vi "handle_kf.vi"(6 "Reset":bool, 7 "Parameters":T2={"Stimulus"={"Type"=enum."Off", "Phase"=0.0, "Amplitude"=[], "Injection point"=enum."Total pose", "Closed loop"=FALSE, "Offset"=[], "Tip -> world"=FALSE, "Frequency"=0.0, "Length"=0.0}, "Goal Filter A"={"Speedup max"=0.0, "Speedup thresh"=0.0, "Speedup nonlin"=0.0, "Filters"=[]}, "Mode controls"={"Hold"=FALSE, "Cancellation"=FALSE, "Goal filter"=FALSE, "Trigger"=FALSE}, "Manipulator type"=enum."Current piezo", "Manipulator calibration"={"Tool offsets"=[[0.0, 0.0, 36200.0]], "Handle light calibration"=[], "Base pivots"=[], "Output pivots"=[], "Length center"=0.0, "Workspace height"=[], "Workspace diameter"=[0.0, 0.0, 36200.0], "Stack travel"=400.0, "Saturation pos"=375.0, "Inverse filters"=[], "Strut length"=0.0}, "Network"={"Remote Host"="", "Send Status"=FALSE, "Send Port"=0, "Recv Commands"=FALSE, "Recv Port"=0}, "Goal Filter B"={"Speedup max"=0.0, "Speedup thresh"=0.0, "Speedup nonlin"=0.0, "Filters"=[]}, "Cancellation"={"KP"={"XY"=0.0, "Rxy"=0.0, "Z"=0.0, "Rz"=0.0}, "KI"=0.0, "KD"={"XY"=0.0, "Rxy"=0.0, "Z"=0.0, "Rz"=0.0}, "Max vel"=20.0, "Max acc"=0.001, "Int error limit"=3.0, "RCM gain"=0.0, "Bypass"=FALSE, "Degraded gain"=0.0}, "Transition time"=0.0, "Estimation"={"Link"={"Measure noise"=[], "Process noise"=[], "Alt process noise"=[], "Alt turnoff cycles"=20, "Innovation limit"=[], "Residue threshold"=0.0, "Enable"=FALSE}, "Handle"={"Measure noise"=[], "Process noise"=[], "State limits"=[], "Innovation limit"=[], "Prediction Lookahead"=0.0, "Enable"=FALSE}}} {"Transition time" format="%_3f"; "Cancellation"."Degraded gain" min=0 max=1 step=0.1 format="%#_3p"; "Cancellation"."RCM gain" min=0 max=1 step=0.1 format="%#_3p"; "Cancellation"."KD"."Rz" min=-1 max=1 step=0.01 format="%#_3p"; "Cancellation"."KD"."Rxy" min=-1 max=1 step=0.01 format="%#_3p"; "Cancellation"."KD"."Z" min=-1 max=1 step=0.01 format="%#_3p"; "Cancellation"."KD"."XY" min=-1 max=1 step=0.01 format="%#_3p"; "Cancellation"."KI" min=0 max=1 step=0.01 format="%#_3p"; "Cancellation"."KP"."Rz" min=-1 max=1 step=0.01 format="%#_3p"; "Cancellation"."KP"."Rxy" min=-1 max=1 step=0.01 format="%#_3p"; "Cancellation"."KP"."Z" min=-1 max=1 step=0.01 format="%#_3p"; "Cancellation"."KP"."XY" min=-1 max=1 step=0.01 format="%#_3p"; "Cancellation"."Max acc" format="%#_3p"; "Goal Filter B"."Filters"."V limit range" format="%_3p"; "Goal Filter B"."Filters"."V limit" format="%_3p"; "Goal Filter B"."Filters"."Upper Q" format="%_3f"; "Goal Filter B"."Filters"."Upper Fc" format="%_3p"; "Goal Filter B"."Filters"."Lower Q" format="%_3f"; "Goal Filter B"."Filters"."Scale factor" format="%_3f"; "Goal Filter B"."Filters"."Lower Fc" format="%_3p"; "Goal Filter B"."Speedup nonlin" format="%_3p"; "Goal Filter B"."Speedup thresh" format="%_3p"; "Goal Filter B"."Speedup max" format="%_3p"; "Manipulator calibration"."Strut length" format="%#_4p"; "Manipulator calibration"."Saturation pos" format="%#.1f"; "Manipulator calibration"."Stack travel" format="%#.1f"; "Manipulator calibration"."Length center" format="%#_4p"; "Manipulator calibration"."Output pivots" format="%#_6f"; "Manipulator calibration"."Base pivots" format="%#_6f"; "Manipulator calibration"."Handle light calibration" format="%#.1f"; "Goal Filter A"."Filters"."V limit range" format="%_3p"; "Goal Filter A"."Filters"."V limit" format="%_3p"; "Goal Filter A"."Filters"."Upper Q" format="%_3f"; "Goal Filter A"."Filters"."Upper Fc" format="%_3p"; "Goal Filter A"."Filters"."Lower Q" format="%_3f"; "Goal Filter A"."Filters"."Scale factor" format="%_3f"; "Goal Filter A"."Filters"."Lower Fc" format="%_3p"; "Goal Filter A"."Speedup nonlin" format="%_3p"; "Goal Filter A"."Speedup thresh" format="%_3p"; "Goal Filter A"."Speedup max" format="%_3p"; "Stimulus"."Length" min=0.0 max=100.0 step=100.0 format="%#_4p"; "Stimulus"."Frequency" min=0.0 step=100.0 format="%#_4g"; "Stimulus"."Offset" format="%#_3p"; "Stimulus"."Amplitude" format="%#_3p"; "Stimulus"."Phase" min=-180.0 max=360.0 step=100.0 format="%#.2f"}, 11 "Handle Pose":T1) -> (1 "Handle State":sgl[][](array[numeric]), 2 "Predicted Handle Pose":T1, 3 "Handle Pose (KF)":T1)   [LabVIEW 2014]
uses:
  utilities/labview/kalman_filter.ctl
  <vilib>/Analysis/Matrix/Datatypes/RealMatrix.ctl
  testing/Micron params.ctl
  testing/stimulus.ctl
  testing/injection_point.ctl
  filtering/goal_loop_parms.ctl
  testing/mode_conrols.ctl
  testing/manipulator_cal.ctl
  asap/labview/testing/probe_calibration.ctl
  host/network_params.ctl
  sq_control_params.ctl
  decoupled_gain.ctl
  estimation_controls.ctl
  utilities/labview/make_trans_mat.vi
  <vilib>/Analysis/Matrix/Numeric/Conversions/Array To Matrix - RA.vi
  utilities/labview/euler_to_rotation.vi
  <vilib>/Analysis/Matrix/NI_Matrix.lvlib
panel:
  in  "Translation filter":T13={"A"=[], "B"=[], "H"=[], "Q"=[], "R"=[], "x"=[], "P"=[], "x lim"=[], "y lim"=[], "K"=[], "Converge count"=-1} {"K" format="%#_3g"; "y lim" format="%#_3g"; "x lim" format="%#_3g"; "P" format="%#_3g"; "H" format="%#_3g"; "x" format="%#_3g"; "Q" format="%#_3g"; "R" format="%#_3g"; "B" format="%#_3g"; "A" format="%#_3g"}
  in  "Rotation filter":T13={"A"=[], "B"=[], "H"=[], "Q"=[], "R"=[], "x"=[], "P"=[], "x lim"=[], "y lim"=[], "K"=[], "Converge count"=-1} {"K" format="%#_3g"; "y lim" format="%#_3g"; "x lim" format="%#_3g"; "P" format="%#_3g"; "H" format="%#_3g"; "x" format="%#_3g"; "Q" format="%#_3g"; "R" format="%#_3g"; "B" format="%#_3g"; "A" format="%#_3g"}
  # "Local variables:"
  # "Position XYZ (microns)"
  # "Velocity XYZ (mm/sec)"
  # "Acceleration XYZ (m/sec)"
  # "Euler angles (radians)"
  # "Euler rates (radians/sec)"
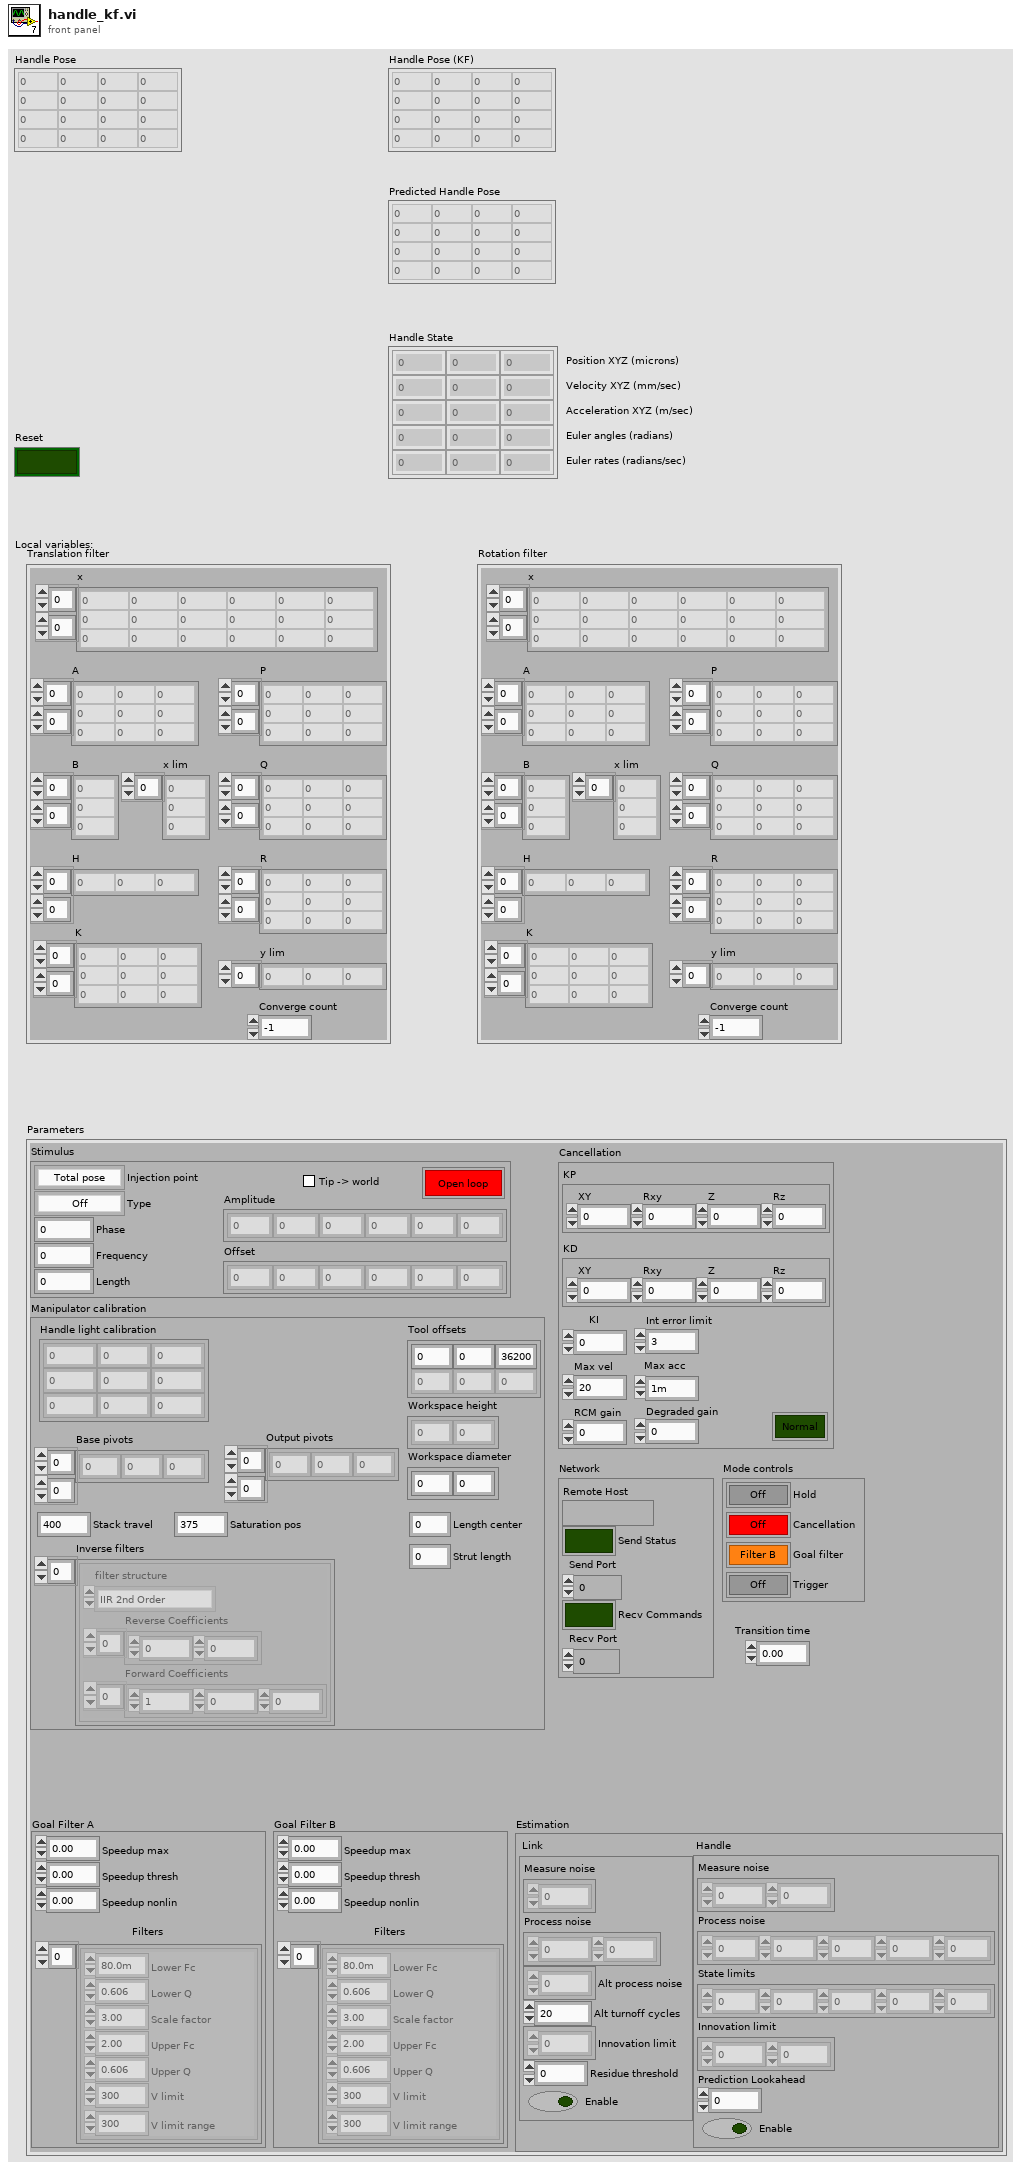
[diagram p1: front panel]
types:
  T1 = typedef "NI_Matrix.lvlib/RealMatrix.ctl" = dbl[][]
  T2 = typedef "Micron params.ctl" = cluster{"Stimulus":T3, "Goal Filter A":T5, "Mode controls":T6, "Manipulator type":enum16{"Current piezo", "Voltage piezo"}, "Manipulator calibration":T7, "Network":T9, "Goal Filter B":T5, "Cancellation":T10, "Transition time":sgl, "Estimation":T12}
  T3 = typedef "stimulus.ctl" = cluster{"Type":enum16{"Off", "Step", "Sine", "Triangle", "Arbitrary"}, "Phase":dbl, "Amplitude":sgl[], "Injection point":T4, "Closed loop":bool, "Offset":sgl[], "Tip -> world":bool, "Frequency":dbl, "Length":dbl}
  T4 = typedef "injection_point.ctl" = enum16{"Total pose", "V limiter", "Goal ", "Link position", "KF link position", "Inverse kin", "Link goal", "Link error", "Controller", "Output", "Drive", "Light"}
  T5 = typedef "goal_loop_parms.ctl" = cluster{"Speedup max":sgl, "Speedup thresh":sgl, "Speedup nonlin":sgl, "Filters":cluster{"Lower Fc":sgl, "Lower Q":sgl, "Scale factor":sgl, "Upper Fc":sgl, "Upper Q":sgl, "V limit":sgl, "V limit range":sgl}[]}
  T6 = typedef "mode_conrols.ctl" = cluster{"Hold":bool, "Cancellation":bool, "Goal filter":bool, "Trigger":bool}
  T7 = typedef "manipulator_cal.ctl" = cluster{"Tool offsets":sgl[][], "Handle light calibration":T8, "Base pivots":sgl[][], "Output pivots":sgl[][], "Length center":sgl, "Workspace height":sgl[], "Workspace diameter":sgl[], "Stack travel":sgl, "Saturation pos":sgl, "Inverse filters":cluster{"filter structure":enum32{"IIR 2nd Order", "IIR 4th Order"}, "Reverse Coefficients":dbl[], "Forward Coefficients":dbl[]}[], "Strut length":sgl}
  T8 = typedef "probe_calibration.ctl" = sgl[][]
  T9 = typedef "network_params.ctl" = cluster{"Remote Host":string, "Send Status":bool, "Send Port":u16, "Recv Commands":bool, "Recv Port":u16}
  T10 = typedef "sq_control_params.ctl" = cluster{"KP":T11, "KI":sgl, "KD":T11, "Max vel":sgl, "Max acc":sgl, "Int error limit":sgl, "RCM gain":sgl, "Bypass":bool, "Degraded gain":sgl}
  T11 = typedef "decoupled_gain.ctl" = cluster{"XY":sgl, "Rxy":sgl, "Z":sgl, "Rz":sgl}
  T12 = typedef "estimation_controls.ctl" = cluster{"Link":cluster{"Measure noise":dbl[], "Process noise":dbl[], "Alt process noise":dbl[], "Alt turnoff cycles":i32, "Innovation limit":dbl[], "Residue threshold":dbl, "Enable":bool}, "Handle":cluster{"Measure noise":dbl[], "Process noise":dbl[], "State limits":dbl[], "Innovation limit":dbl[], "Prediction Lookahead":sgl, "Enable":bool}}
  T13 = typedef "kalman_filter.ctl" = cluster{"A":T1, "B":T1, "H":T1, "Q":T1, "R":T1, "x":T1, "P":T1, "x lim":dbl[], "y lim":dbl[], "K":T1, "Converge count":i32}
  T14 = cluster{"Measure noise":dbl[], "Process noise":dbl[], "State limits":dbl[], "Innovation limit":dbl[], "Prediction Lookahead":sgl, "Enable":bool}
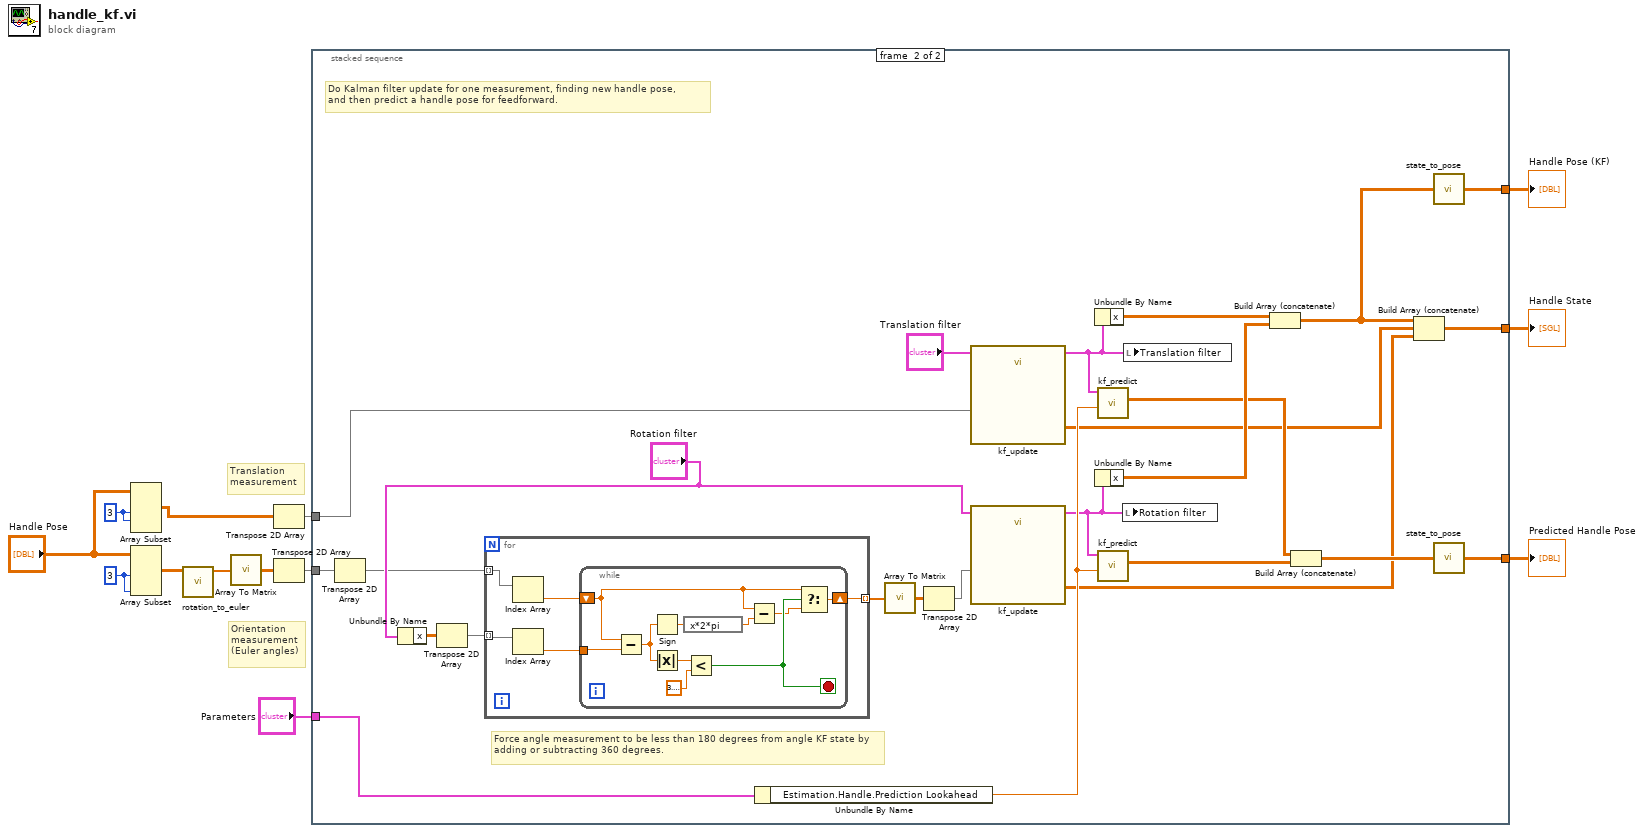
[diagram p0: block diagram]
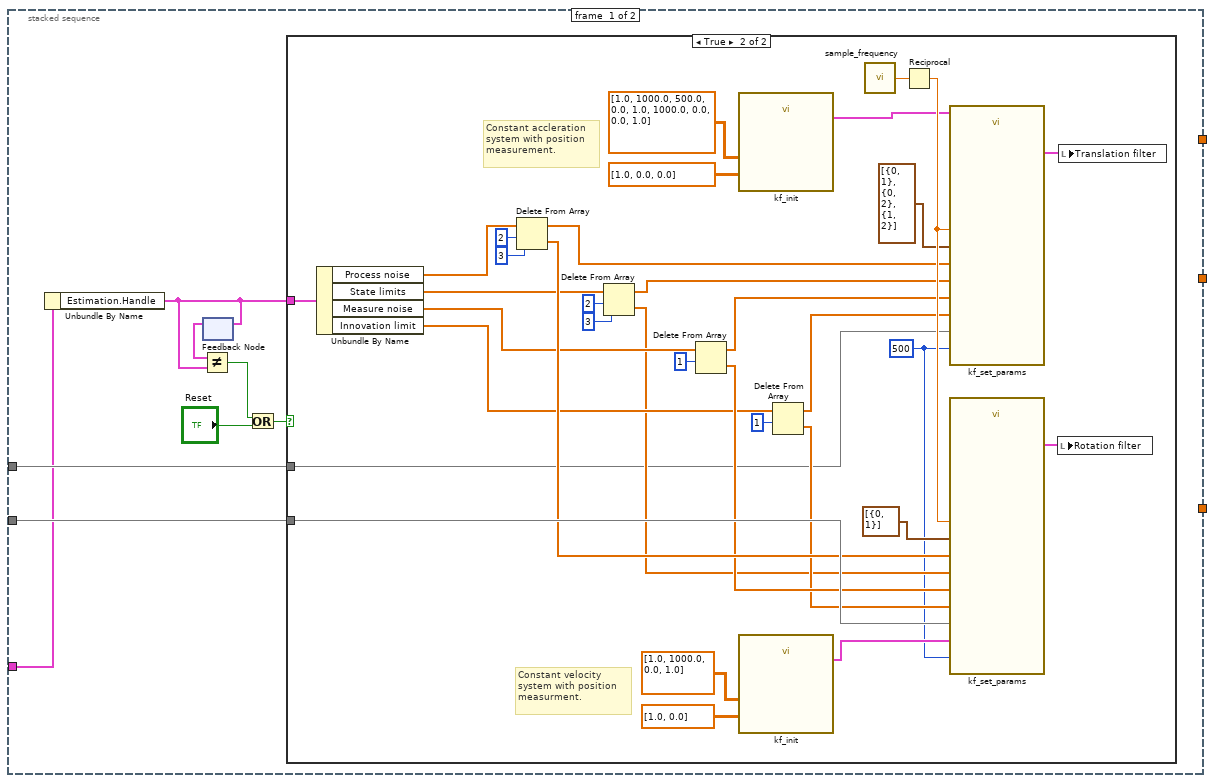
[diagram p2: hidden frame]
diagram:
  w2 = 3 ("length")
  w12 = 3 ("length")
  # "Orientation\nmeasurement\n(Euler angles)"
  # "Translation\nmeasurement"
  n1 = Array Subset(array="Handle Pose", length (row)=w2, index (col)=w2) -> (w1:T1)  [unwired: 2 in]
  n2 = Array Subset(array="Handle Pose", length (row)=w12, length (col)=w12) -> (w11:T1)  [unwired: 2 in]
  n3 = call "rotation_to_euler.vi"("Rotation"=w11) -> ("Theta XYZ"=w9:dbl[])  [unwired: 10 in]
  n4 = call-poly <vilib>:"Array To Matrix.vi"("Real 1D Array"=w9) -> ("Real Matrix (Column Vector)"=w10:T1)
  n5 = Transpose 2D Array(2D array=w1) -> (transposed array=w13:T1)
  n6 = Transpose 2D Array(2D array=w10) -> (transposed array=w8:T1)
  n7 = stacked-sequence {
    tunnel: w8 -> [w21 w67]
    tunnel: w13 -> [w20 w80]
    tunnel: "Parameters" -> [w19 w76]
    tunnel: [_ w56] -> w7
    tunnel: [_ w72] -> w5
    tunnel: [_ w68] -> w4
    frame #0 {
      n8 = Unbundle By Name(w19) -> ("Estimation.Handle"=w17:T14)
      n9 = feedback-in #1(w17) -> ()
      n10 = feedback #1() -> (w16:T14)  [unwired: 1 in]
      n11 = Not Equal?(x=w16, y=w17) -> (x != y?=w14:bool)
      n12 = Or(x=w14, y="Reset") -> (x .or. y?=w15:bool)
      n13 = case shown="True" w15 {
        tunnel: w17 -> [_ w53]
        tunnel: w21 -> [_ w49]
        tunnel: w20 -> [_ w23]
        frame False {
        }
        frame True {
          w22 = 500 ("Converge count")
          # "Constant velocity system with position measurment."
          # "Constant accleration system with position measurement."
          n14 = Unbundle By Name(w53) -> ("Process noise"=w48:dbl[], "State limits"=w32:dbl[], "Measure noise"=w43:dbl[], "Innovation limit"=w38:dbl[])
          n15 = Delete From Array(array=w48, length=2, index=3) -> (deleted portion=w44:dbl[], array with subset deleted=w45:dbl[])
          n16 = Delete From Array(array=w32, length=2, index=3) -> (deleted portion=w30:dbl[], array with subset deleted=w31:dbl[])
          n17 = Delete From Array(array=w43, length=1) -> (deleted portion=w41:dbl[], array with subset deleted=w42:dbl[])  [unwired: 1 in]
          n18 = call "kf_init.vi"("A"=T1 [[1.0, 1000.0, 500.0], [0.0, 1.0, 1000.0], [0.0, 0.0, 1.0]], "H"=T1 [[1.0, 0.0, 0.0]] ("A")) -> ("KF out"=w27:T13)  [unwired: 13 in]
          n19 = call "kf_init.vi"("A"=T1 [[1.0, 1000.0], [0.0, 1.0]], "H"=T1 [[1.0, 0.0]] ("A")) -> ("KF out"=w24:T13)  [unwired: 13 in]
          n20 = Delete From Array(array=w38, length=1) -> (deleted portion=w36:dbl[], array with subset deleted=w37:dbl[])  [unwired: 1 in]
          n21 = call "sample_frequency.vi"() -> ("Sample frequency"=w55:dbl)
          n22 = Reciprocal(x=w55) -> (1/x=w54:dbl)
          n23 = call "kf_set_params.vi"("KF in"=w27, "State limits"=w31, "Innovation limits"=w37, "Process noise"=w45, "Initial input"=w23, "Measurement noise"=w42, "A scale indices"=cluster{"Row":i32, "Column":i32}[] [{"Row"=0, "Column"=1}, {"Row"=0, "Column"=2}, {"Row"=1, "Column"=2}], "Scale factor"=w54, "Converge count"=w22) -> ("KF out"=w51:T13)  [unwired: 10 in]
          n24 = call "kf_set_params.vi"("KF in"=w24, "State limits"=w30, "Innovation limits"=w36, "Process noise"=w44, "Initial input"=w49, "Measurement noise"=w41, "A scale indices"=cluster{"Row":i32, "Column":i32}[] [{"Row"=0, "Column"=1}], "Scale factor"=w54, "Converge count"=w22) -> ("KF out"=w50:T13)  [unwired: 10 in]
          n25 = local write "Rotation filter"(w50) -> ()
          n26 = local write "Translation filter"(w51) -> ()
        }
      }
    }
    frame #1 {
      # "Force angle measurement to be less than 180 degrees from angle KF state by adding or subtracting 360 degrees."
      # "Do Kalman filter update for one measurement, finding new handle pose,\nand then predict a handle pose for feedforward."
      n27 = Transpose 2D Array(2D array=w67) -> (transposed array=w63:T1)
      n28 = Unbundle By Name("Rotation filter") -> ("x"=w65:T1)
      n29 = Transpose 2D Array(2D array=w65) -> (transposed array=w64:T1)
      n30 = for {
        tunnel: w64 -> [w85] mode=indexing
        tunnel: w63 -> [w84] mode=indexing
        tunnel: [w81] -> w62 mode=indexing
        n31 = Index Array(array=w84) -> (element=w82:dbl)  [unwired: 1 in]
        n32 = Index Array(array=w85) -> (element=w83:dbl)  [unwired: 1 in]
        n33 = while {
          tunnel: w83 -> [w88]
          shift-right: [w92] -> w81
          shift-left: w82 -> [w86]
          stop <- w91 stop-if-true
          n34 = Subtract(x=w86, y=w88) -> (x-y=w93:dbl)
          n35 = Sign(1:w93) -> (0:w90:dbl)
          n36 = Absolute Value(x=w93) -> (abs(x)=w95:dbl)
          n37 = expression code="x*2*pi"(w90) -> (w89:dbl)
          n38 = Less?(x=w95, y=3.141592653589793) -> (x < y?=w91:bool)
          n39 = Subtract(x=w86, y=w89) -> (x-y=w87:dbl)
          n40 = Select(t=w86, s=w91, f=w87) -> (s? t:f=w92:dbl)
        }
      }
      n41 = Unbundle By Name(w76) -> ("Estimation.Handle.Prediction Lookahead"=w75:sgl)
      n42 = call-poly <vilib>:"Array To Matrix.vi"("Real 1D Array"=w62) -> ("Real Matrix (Column Vector)"=w61:T1)
      n43 = Transpose 2D Array(2D array=w61) -> (transposed array=w60:T1)
      n44 = call "kf_update.vi"("z"=w80, "KF in"="Translation filter") -> ("y"=w58:T1, "KF out"=w73:T13)  [unwired: 8 in]
      n45 = call "kf_update.vi"("z"=w60, "KF in"="Rotation filter") -> ("y"=w57:T1, "KF out"=w74:T13)  [unwired: 8 in]
      n46 = Unbundle By Name(w73) -> ("x"=w78:T1)
      n47 = Unbundle By Name(w74) -> ("x"=w77:T1)
      n48 = call "kf_predict.vi"("Steps"=w75, "KF in"=w73) -> ("Predicted state"=w71:T1)  [unwired: 9 in]
      n49 = call "kf_predict.vi"("Steps"=w75, "KF in"=w74) -> ("Predicted state"=w70:T1)  [unwired: 9 in]
      n50 = local write "Rotation filter"(w74) -> ()
      n51 = local write "Translation filter"(w73) -> ()
      n52 = Build Array (concatenate)(w78, w77) -> (w59:T1)
      n53 = Build Array (concatenate)(w71, w70) -> (w69:T1)
      n54 = Build Array (concatenate)(w59, w58, w57) -> (w56:T1)
      n55 = call "state_to_pose.vi"("Handle State"=w59) -> ("Pose"=w72:T1)
      n56 = call "state_to_pose.vi"("Handle State"=w69) -> ("Pose"=w68:T1)
    }
  }
  "Handle Pose (KF)" <- w5
  "Handle State" <- w7
  "Predicted Handle Pose" <- w4
